vi "Swerve ShouldReverse.vi"(9 "ca in":dbl, 10 "wa in":dbl) -> (2 "shouldReverse out":bool)   [LabVIEW 2018]
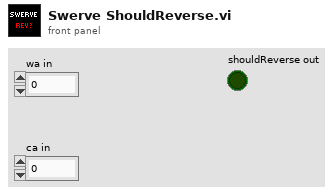
[diagram p1: front panel]
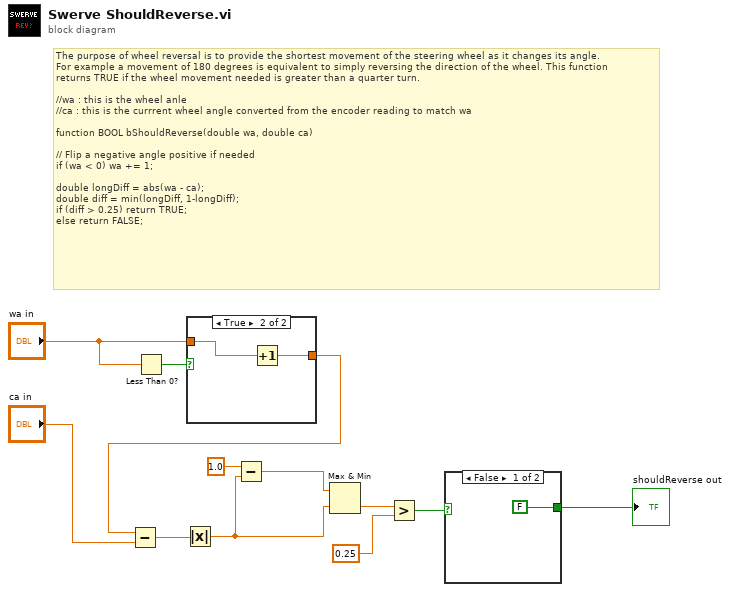
[diagram p0: block diagram]
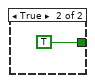
[diagram p2: hidden frame]
diagram:
  # "The purpose of wheel reversal is to provide the shortest movement of the steering wheel as it changes its angle.\nFor example a movement of 180 degrees is equivalent to simply reversing the direction of the wheel. This function \nreturns TRUE if the wheel movement needed is greater than a quarter turn.\n\n//wa : this is the wheel anle\n//ca : this is the currrent wheel angle converted from the encoder reading to match wa\n\nfunction BOOL bShouldReverse(double wa, double ca)\n\n// Flip a negative angle positive if needed\nif (wa < 0) wa += 1;\n\ndouble longDiff = abs(wa - ca);\ndouble diff = min(longDiff, 1-longDiff);\nif (diff > 0.25) return TRUE;\nelse return FALSE;"
  n1 = Less Than 0?(x="wa in") -> (x < 0?=w12:bool)
  n2 = case shown="True" w12 {
    tunnel: "wa in" -> [w13 w15]
    tunnel: [w13 w14] -> w1
    frame False {
    }
    frame True {
      n3 = Increment(x=w15) -> (x+1=w14:dbl)
    }
  }
  n4 = Subtract(x=w1, y="ca in") -> (x-y=w9:dbl)
  n5 = Absolute Value(x=w9) -> (abs(x)=w6:dbl)
  n6 = Subtract(x=1.0, y=w6) -> (x-y=w7:dbl)
  n7 = Max & Min(x=w7, y=w6) -> (min(x,y)=w5:dbl)  [unwired: 1 out]
  n8 = Greater?(x=w5, y=0.25) -> (0:w3:bool)
  n9 = case shown="False" w3 {
    tunnel: [FALSE TRUE] -> w2
    frame False {
    }
    frame True {
    }
  }
  "shouldReverse out" <- w2
